vi "Entry Console - Fire Steps.vi"(8 "error in (no error)":errorcluster, 9 "CarWash States":T1, 10 "Entry Console Data":T2, 11 "View Model":T3) -> (0 "error out":errorcluster, 3 "View Model":T3)   [LabVIEW 2017]
doc: "Generates user event with variant data when state is changed"
uses:
  View Model/Controls/View Model.ctl
  Configuration Database/Controls/Config Model.ctl
  Configuration Database/Controls/Congif Data.ctl
  Configuration Database/Controls/Config Commands.ctl
  View Model/Controls/Shared Model.ctl
  Error Handler/Controls/Error Model.ctl
  Error Handler/Controls/Error Data.ctl
  Error Handler/Controls/Error Type.ctl
  Car Wash Controller/Controls/Car Wash Model.ctl
  Car Wash Controller/Controls/Car Wash States.ctl
  Car Wash Controller/Controls/Controller Overhead.ctl
  Car Wash Controller/Controls/Vehicle Location.ctl
  Car Wash Controller/Controls/CarWash CMD.ctl
  Controls/Entry Console Data.ctl
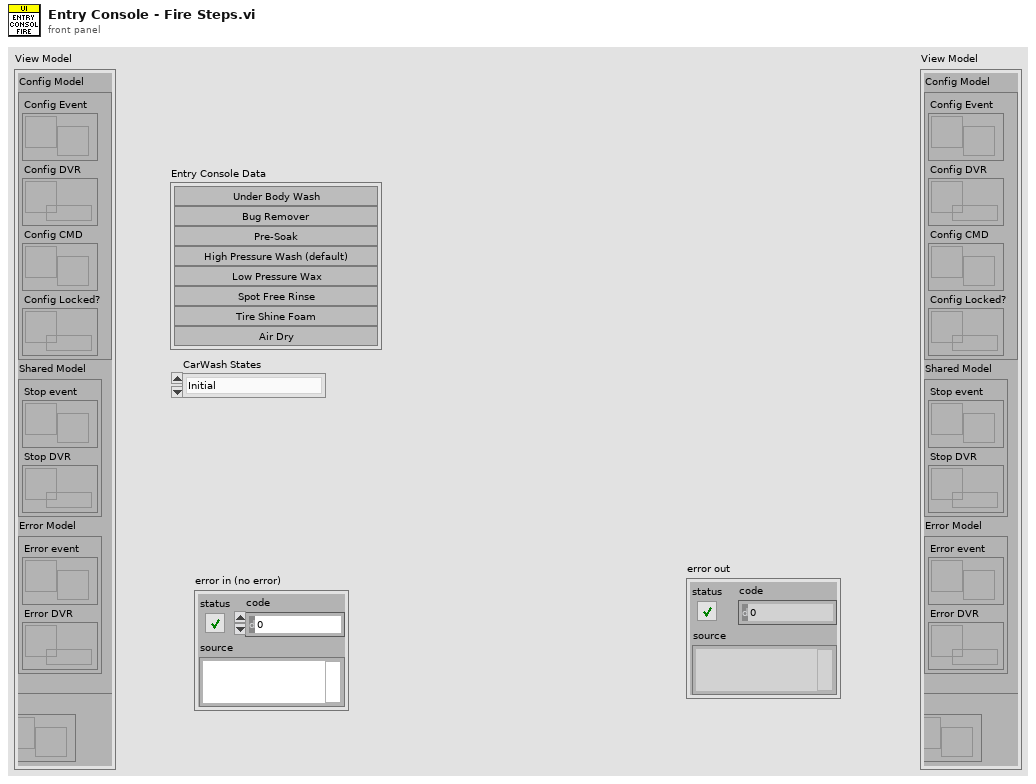
[diagram p1: front panel]
types:
  T1 = typedef "Car Wash States.ctl" = enum16{"Initial", "Wait for start", "Start", "Wait for vehicle", "Wash Step Execution", "Wash Step Complete", "Wash Cycle Complete", "Wash Exit", "Wash Abort", "Terminate"}
  T2 = typedef "Entry Console Data.ctl" = cluster{"Under Body Wash":bool, "Bug Remover":bool, "Pre-Soak":bool, "High Pressure Wash":bool, "Low Pressure Wax":bool, "Spot Free Rinse":bool, "Tire Shine Foam":bool, "Air Dry":bool}
  T3 = typedef "View Model.ctl" = cluster{"Config Model":T4, "Shared Model":T5, "Error Model":T6, "Car Wash Model":T7}
  T4 = typedef "Config Model.ctl" = cluster{"Config Event":refnum<user-event>, "Config DVR":refnum<data-value>, "Config CMD":refnum<user-event>, "Config Locked?":refnum<data-value>}
  T5 = typedef "Shared Model.ctl" = cluster{"Stop event":refnum<user-event>, "Stop DVR":refnum<data-value>}
  T6 = typedef "Error Model.ctl" = cluster{"Error event":refnum<user-event>, "Error DVR":refnum<data-value>}
  T7 = typedef "Car Wash Model.ctl" = cluster{"State Change":refnum<user-event>, "Out of Position Change":refnum<user-event>, "Wash Entry Change":refnum<user-event>, "Contr Overhead DVR":refnum<data-value>, "Contr Overhead Event":refnum<user-event>, "CarWash CMD":refnum<user-event>, "Location Change":refnum<user-event>}
  T8 = typedef "CarWash CMD.ctl" = cluster{"CarWash States":T1, "Variant":variant}
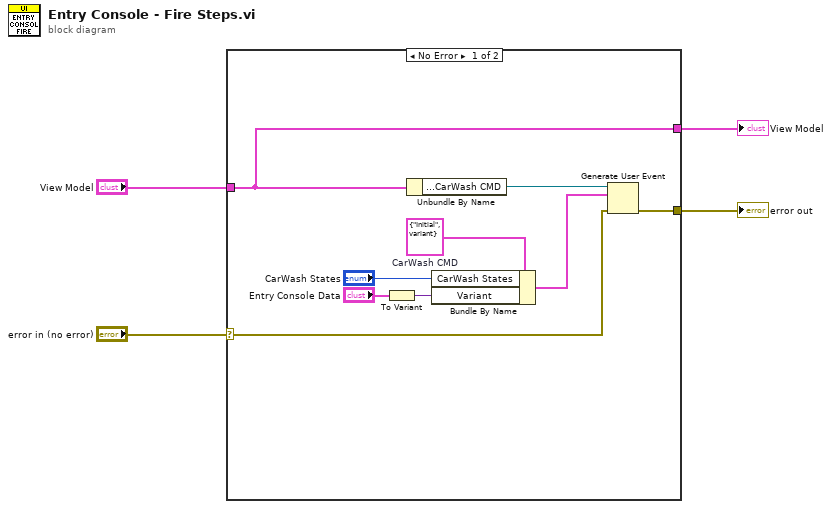
[diagram p0: block diagram]
diagram:
  n1 = case shown="No Error" "error in (no error)" {
    selector: "error in (no error)" -> [w11 w14]
    tunnel: "View Model" -> [w13 w15]
    tunnel: [w13 w15] -> w2
    tunnel: [w12 w14] -> w1
    frame No Error {
      w9 = T8 {"CarWash States"=enum."Initial", "Variant"=variant}  # CarWash CMD
      n2 = To Variant(anything="Entry Console Data") -> (Variant=w5:variant)
      n3 = Unbundle By Name(w13) -> ("Car Wash Model.CarWash CMD"=w10:refnum<user-event>)
      n4 = Bundle By Name(cluster=w9, "CarWash States"="CarWash States", "Variant"=w5) -> (w8:T8)
      n5 = Generate User Event(user event=w10, event data cluster=w8, error in=w11) -> (error out=w12:errorcluster)  [unwired: 1 in, 1 out]
    }
    frame Error {
    }
  }
  "View Model" <- w2
  "error out" <- w1
